vi "Set Time.vi"() -> ()   [LabVIEW 2020]
panel:
  out "Start Time":dbl[][](array[numeric])
  out "End Time":dbl[][](array[numeric])
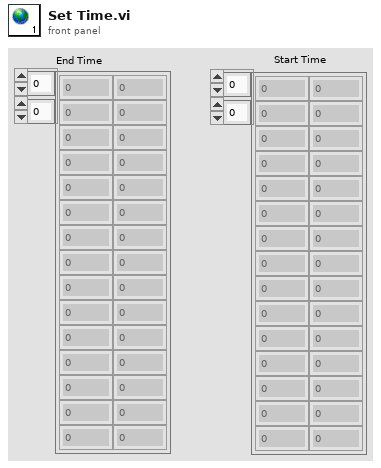
[diagram p1: front panel]
diagram:
